vi "DefenderNormal.vi"(1 "Atacando contra?":bool=TRUE, 3 "AI Parameters":T1={"GotoKick"={"Dist do cone a frente"=150.0, "attacker farback"=1500.0, "Perto"=300.0, "min dist to kick"=150.0, "kick eps"=0.05, "Time to transition"=0.0}, "Attacker"={"CC chute"=0.09, "CC passe"=0.045, "Kick Force"=100.0, "D ball-robot Kick"=200.0, "D ball-robot Pass"=0.3}, "Defender"={"D max"=1700.0, "Vel p/ robô av"=1000.0, "Kick Force"=100.0, "D atk-def"=0.0, "D farback"=0.0}, "Timeout"={"Field/v in x"=6.0, "Dist Robots"=300, "Dist up in y"=300}, "Pose Striker"={"dist"=200.0, "Numeric"=-4.0, "dist 2"=200.0}, "Dist Stop"=300.0, "Distance when ball out"=200, "D central gap "=150.0, "T pass"=0.0, "Force ++"=0.0, "range kick"=0.0} {"D central gap" format="%#_13g"; "Dist Stop" format="%#_13g"; "Pose Striker"."Numeric" format="%#_13g"; "Defender"."Kick Force" format="%#_13g"; "Defender"."Vel p/ robô av" format="%#_13g"; "Attacker"."D ball-robot Kick" format="%#_13g"; "Attacker"."Kick Force" format="%#_13g"; "Attacker"."CC passe" format="%#_13g"; "Attacker"."CC chute" format="%#_13g"; "GotoKick"."kick eps" format="%#_13g"; "GotoKick"."min dist to kick" format="%#_13g"; "GotoKick"."Perto" format="%#_13g"; "GotoKick"."attacker farback" format="%#_13g"; "GotoKick"."Dist do cone a frente" format="%#_13g"}, 4 "IA State Input 2":T2={"our_robots"=[], "enemy_robots"=[], "balls"=[], "geometry"={"line_width"=0, "field_length"=0, "field_width"=0, "boundary_width"=0, "referee_width"=0, "goal_width"=0, "goal_depth"=0, "goal_wall_width"=0, "center_circle_radius"=0, "defense_radius"=0, "defense_stretch"=0, "free_kick_from_defense_dist"=0, "penalty_spot_from_field_line_dist"=0, "penalty_line_from_spot_dist"=0}, "IA Judge"={"stage"="", "command"="", "our_goalie_id"=0.0, "enemy_goalie_id"=0.0, "command enum"=enum."Halt", "Time"=enum."Azul"}, "Received Timestamp"=timestamp(0 s since 1904-01-01), "Events"={"Touch"=FALSE, "Ball out"=FALSE, "id touch"=0.0, "Ball out of \nVision"=FALSE, "Ball inside \nGoalie area"=FALSE, "Robot not responding"=FALSE, "Robots responding status"=[1.0, 1.0, 1.0, 1.0, 1.0, 1.0], "Enemy Ball \nPossession"=FALSE, "Pass State"=FALSE, "id end of pass"=0.0, "Kick"=FALSE, "Id ini Possession"=0.0, "Ball Possesion"=FALSE, "Id Possesion"=0.0}}, 5 "Stop?":bool, 6 "Defensores":u32[](array[numeric]), 7 "total":i32, 8 "Field defense":dbl[](array[numeric]), 9 "Field Size in":T7, 10 "balls":T6[](array[typedef]), 11 "Our Robot in":T3={"id"=0, "function"=enum."Attacker", "x"=0.0, "y"=0.0, "orientation"=0.0, "v_tangent"=0.0, "v_normal"=0.0, "v_ang"=0.0, "kick_x"=0.0, "kick_z"=0.0, "dribble"=FALSE, "Timestamp"=timestamp(0 s since 1904-01-01), "dest_x"=0.0, "dest_y"=0.0, "dest_orientation"=0.0, "estimatives"={"est_v_tangent"=0.0, "est_v_normal"=0.0, "est_vx"=0.0, "est_vy"=0.0, "Pos Robot Est"=[]}, "dest_x_kick"=0.0, "dest_y_kick"=0.0, "Gap Coord"=[], "States"=enum."GoToTangent"}) -> (2 "Robot out":T3={"id"=0, "function"=enum."Attacker", "x"=0.0, "y"=0.0, "orientation"=0.0, "v_tangent"=0.0, "v_normal"=0.0, "v_ang"=0.0, "kick_x"=0.0, "kick_z"=0.0, "dribble"=FALSE, "Timestamp"=timestamp(0 s since 1904-01-01), "dest_x"=0.0, "dest_y"=0.0, "dest_orientation"=0.0, "estimatives"={"est_v_tangent"=0.0, "est_v_normal"=0.0, "est_vx"=0.0, "est_vy"=0.0, "Pos Robot Est"=[]}, "dest_x_kick"=0.0, "dest_y_kick"=0.0, "Gap Coord"=[], "States"=enum."GoToTangent"})   [LabVIEW 2016]
uses:
  Core/AI Robot.ctl
  Functions Enum.ctl
  AttackerStates.ctl
  Core/AI Ball.ctl
  Core/Field Size.ctl
  Core/AI Input.ctl
  Core/AI Judge.ctl
  Command Enum.ctl
  Util/Events/Events.ctl
  AI Parameters.ctl
  <vilib>/Analysis/_algsub.llb/Real Vector Norm.vi
  <vilib>/Analysis/NI_AALPro.lvlib
panel:
  in  "element":dbl=-2000.0 format="%#_13g"
  in  "dist to defender\nattacker evasion":dbl=200.0
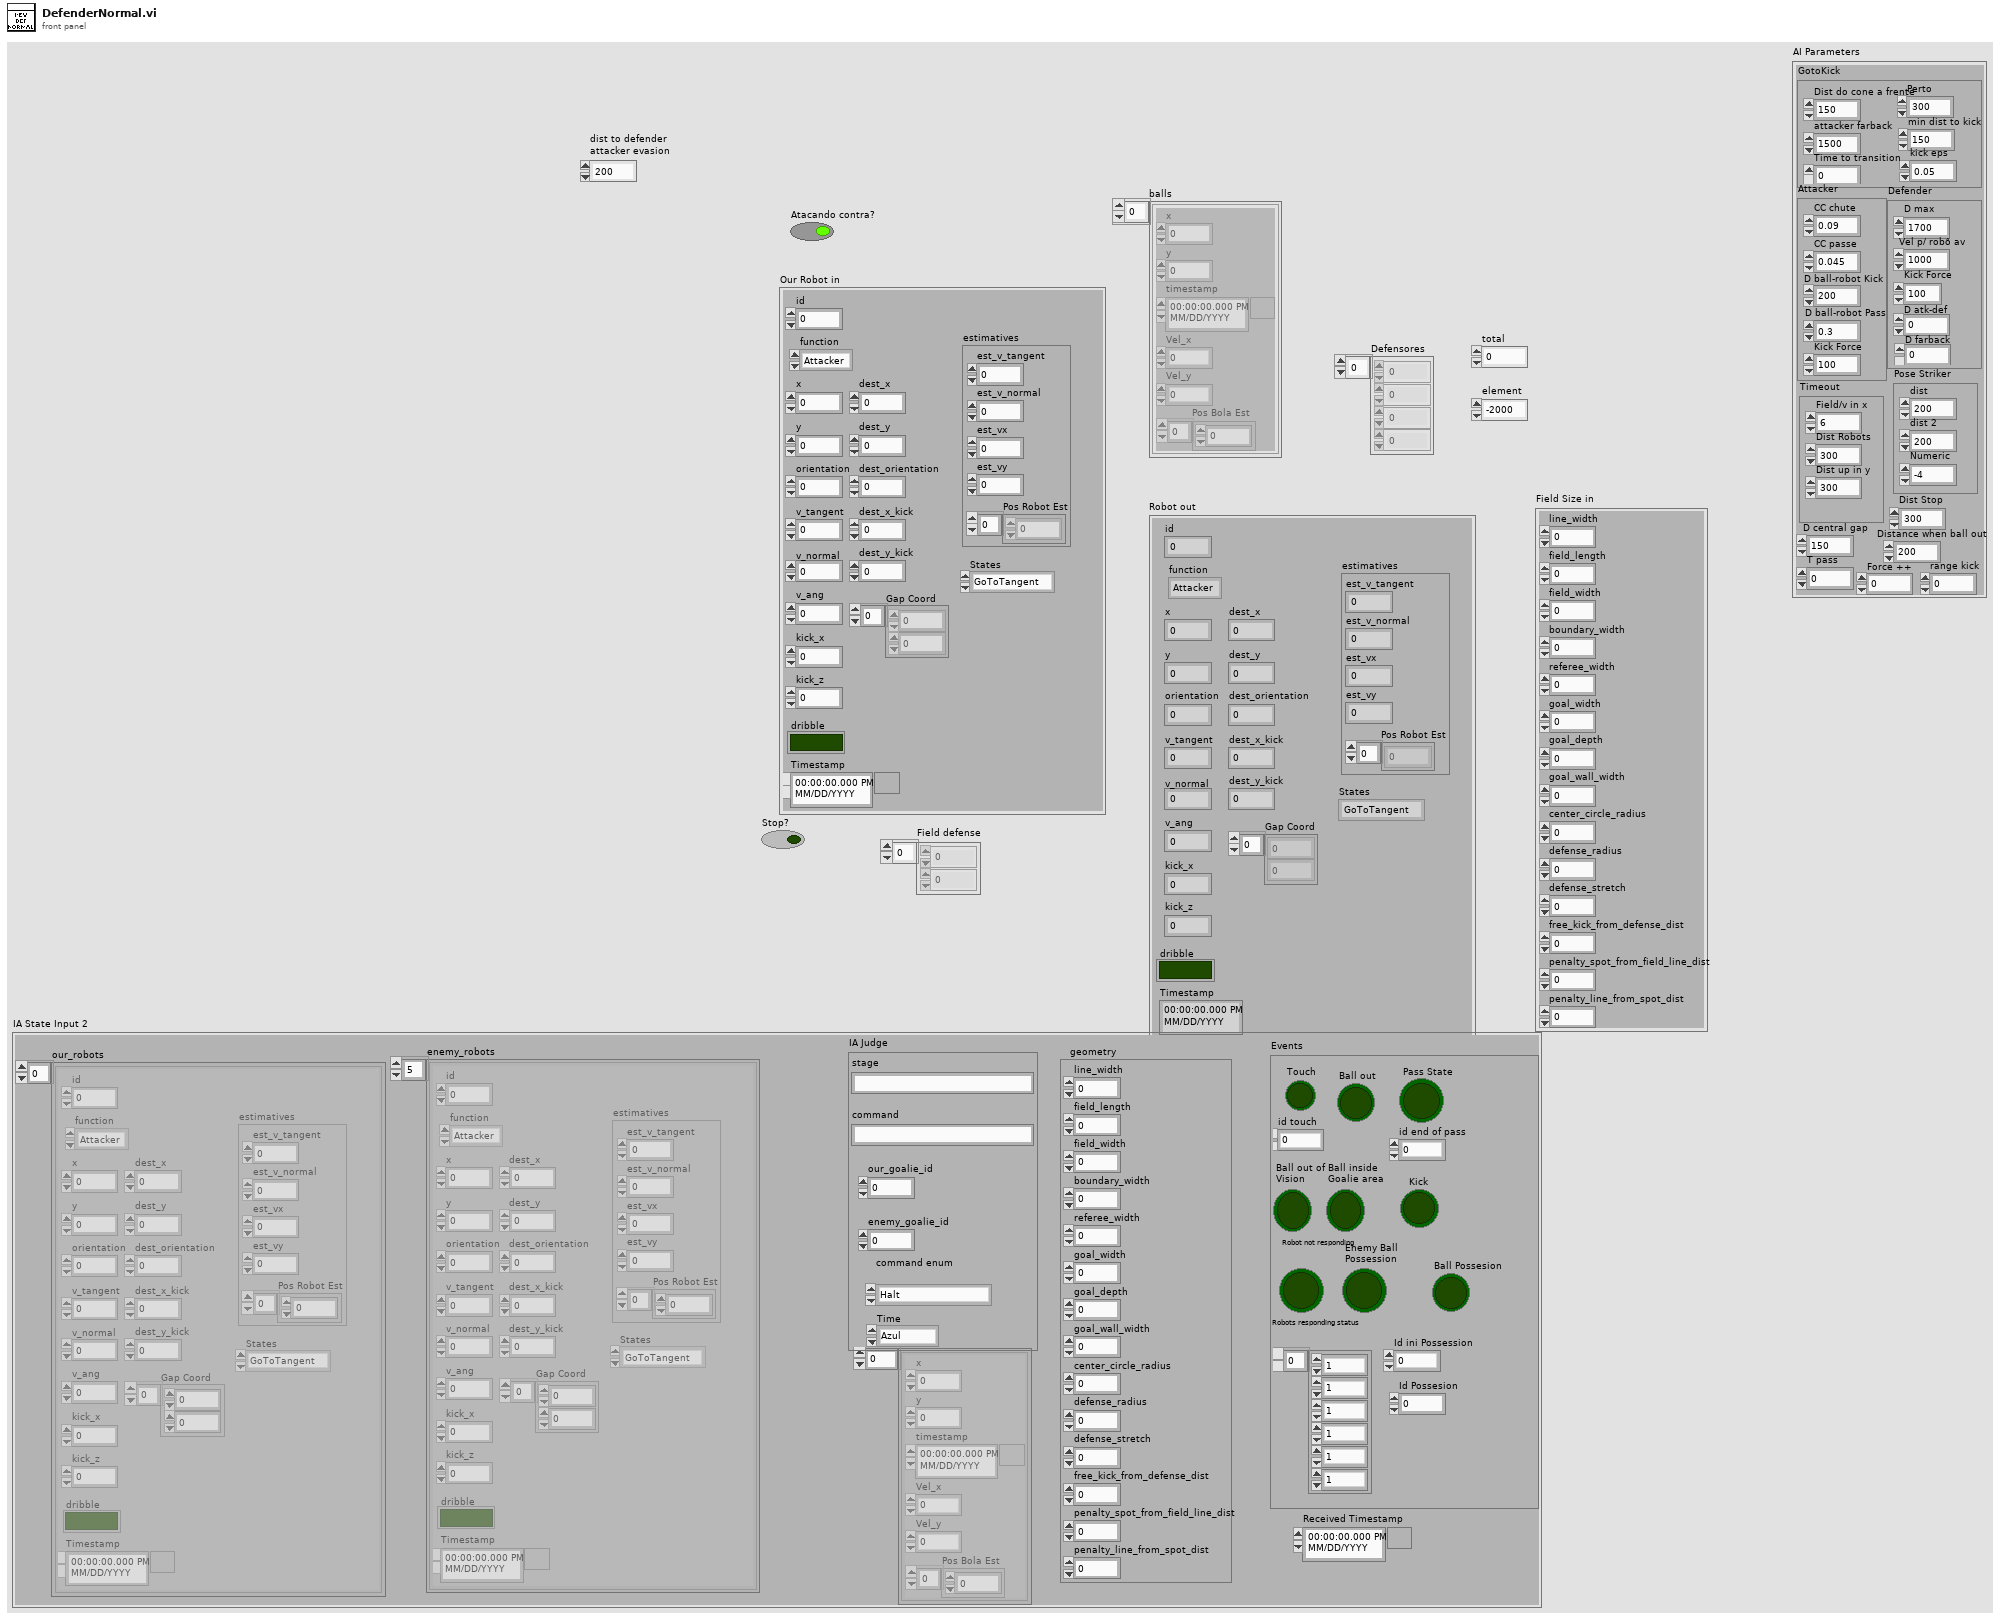
[diagram p1: front panel]
types:
  T1 = typedef "AI Parameters.ctl" = cluster{"GotoKick":cluster{"Dist do cone a frente":dbl, "attacker farback":dbl, "Perto":dbl, "min dist to kick":dbl, "kick eps":dbl, "Time to transition":dbl}, "Attacker":cluster{"CC chute":dbl, "CC passe":dbl, "Kick Force":dbl, "D ball-robot Kick":dbl, "D ball-robot Pass":dbl}, "Defender":cluster{"D max":dbl, "Vel p/ robô av":dbl, "Kick Force":dbl, "D atk-def":dbl, "D farback":dbl}, "Timeout":cluster{"Field/v in x":dbl, "Dist Robots":u32, "Dist up in y":u32}, "Pose Striker":cluster{"dist":dbl, "Numeric":dbl, "dist 2":dbl}, "Dist Stop":dbl, "Distance when ball out":i32, "D central gap ":dbl, "T pass":dbl, "Force ++":dbl, "range kick":dbl}
  T2 = typedef "AI Input.ctl" = cluster{"our_robots":T3[], "enemy_robots":T3[], "balls":T6[], "geometry":T7, "IA Judge":T8, "Received Timestamp":timestamp, "Events":T10}
  T3 = typedef "AI Robot.ctl" = cluster{"id":u32, "function":T4, "x":dbl, "y":dbl, "orientation":dbl, "v_tangent":dbl, "v_normal":dbl, "v_ang":dbl, "kick_x":dbl, "kick_z":dbl, "dribble":bool, "Timestamp":timestamp, "dest_x":dbl, "dest_y":dbl, "dest_orientation":dbl, "estimatives":cluster{"est_v_tangent":dbl, "est_v_normal":dbl, "est_vx":dbl, "est_vy":dbl, "Pos Robot Est":dbl[]}, "dest_x_kick":dbl, "dest_y_kick":dbl, "Gap Coord":dbl[], "States":T5}
  T4 = typedef "Functions Enum.ctl" = enum16{"Attacker", "Goalie", "Defender", "Striker", "Goto 0", "Dummy", "Kicker", "ZigZag"}
  T5 = typedef "AttackerStates.ctl" = enum16{"Pass", "GoToTangent", "BallGetting", "GoToKick", ""}
  T6 = typedef "AI Ball.ctl" = cluster{"x":dbl, "y":dbl, "timestamp":timestamp, "Vel_x":dbl, "Vel_y":dbl, "Pos Bola Est":dbl[]}
  T7 = typedef "Field Size.ctl" = cluster{"line_width":u32, "field_length":u32, "field_width":u32, "boundary_width":u32, "referee_width":u32, "goal_width":u32, "goal_depth":u32, "goal_wall_width":u32, "center_circle_radius":u32, "defense_radius":u32, "defense_stretch":u32, "free_kick_from_defense_dist":u32, "penalty_spot_from_field_line_dist":u32, "penalty_line_from_spot_dist":u32}
  T8 = typedef "AI Judge.ctl" = cluster{"stage":string, "command":string, "our_goalie_id":dbl, "enemy_goalie_id":dbl, "command enum":T9, "Time":enum16{"Azul", "Amarelo"}}
  T9 = typedef "Command Enum.ctl" = enum16{"Halt", "Stop", "Force Start", "PKA Normal Start", "Prepare Kickoff Ally", "PKE Normal Start", "Prepare Kickoff Enemy", "Prepare Penalty Ally", "PPA Normal Start", "Prepare Penalty Enemy", "PPE Normal Start", "Direct Free Enemy", "Direct Free Ally", "Indirect Free Enemy", "Indirect Free Ally", "Timeout Enemy", "Timeout Ally", "Goal Enemy", "Goal Ally", "Ball Placement Enemy", "Ball Placement Ally", "Normal Half Time", "Extra Time Break", "Extra Half Time", "None", "Post Game"}
  T10 = typedef "Events.ctl" = cluster{"Touch":bool, "Ball out":bool, "id touch":dbl, "Ball out of \nVision":bool, "Ball inside \nGoalie area":bool, "Robot not responding":bool, "Robots responding status":dbl[], "Enemy Ball \nPossession":bool, "Pass State":bool, "id end of pass":dbl, "Kick":bool, "Id ini Possession":dbl, "Ball Possesion":bool, "Id Possesion":dbl}
  T11 = cluster{"D max":dbl, "Vel p/ robô av":dbl, "Kick Force":dbl, "D atk-def":dbl, "D farback":dbl}
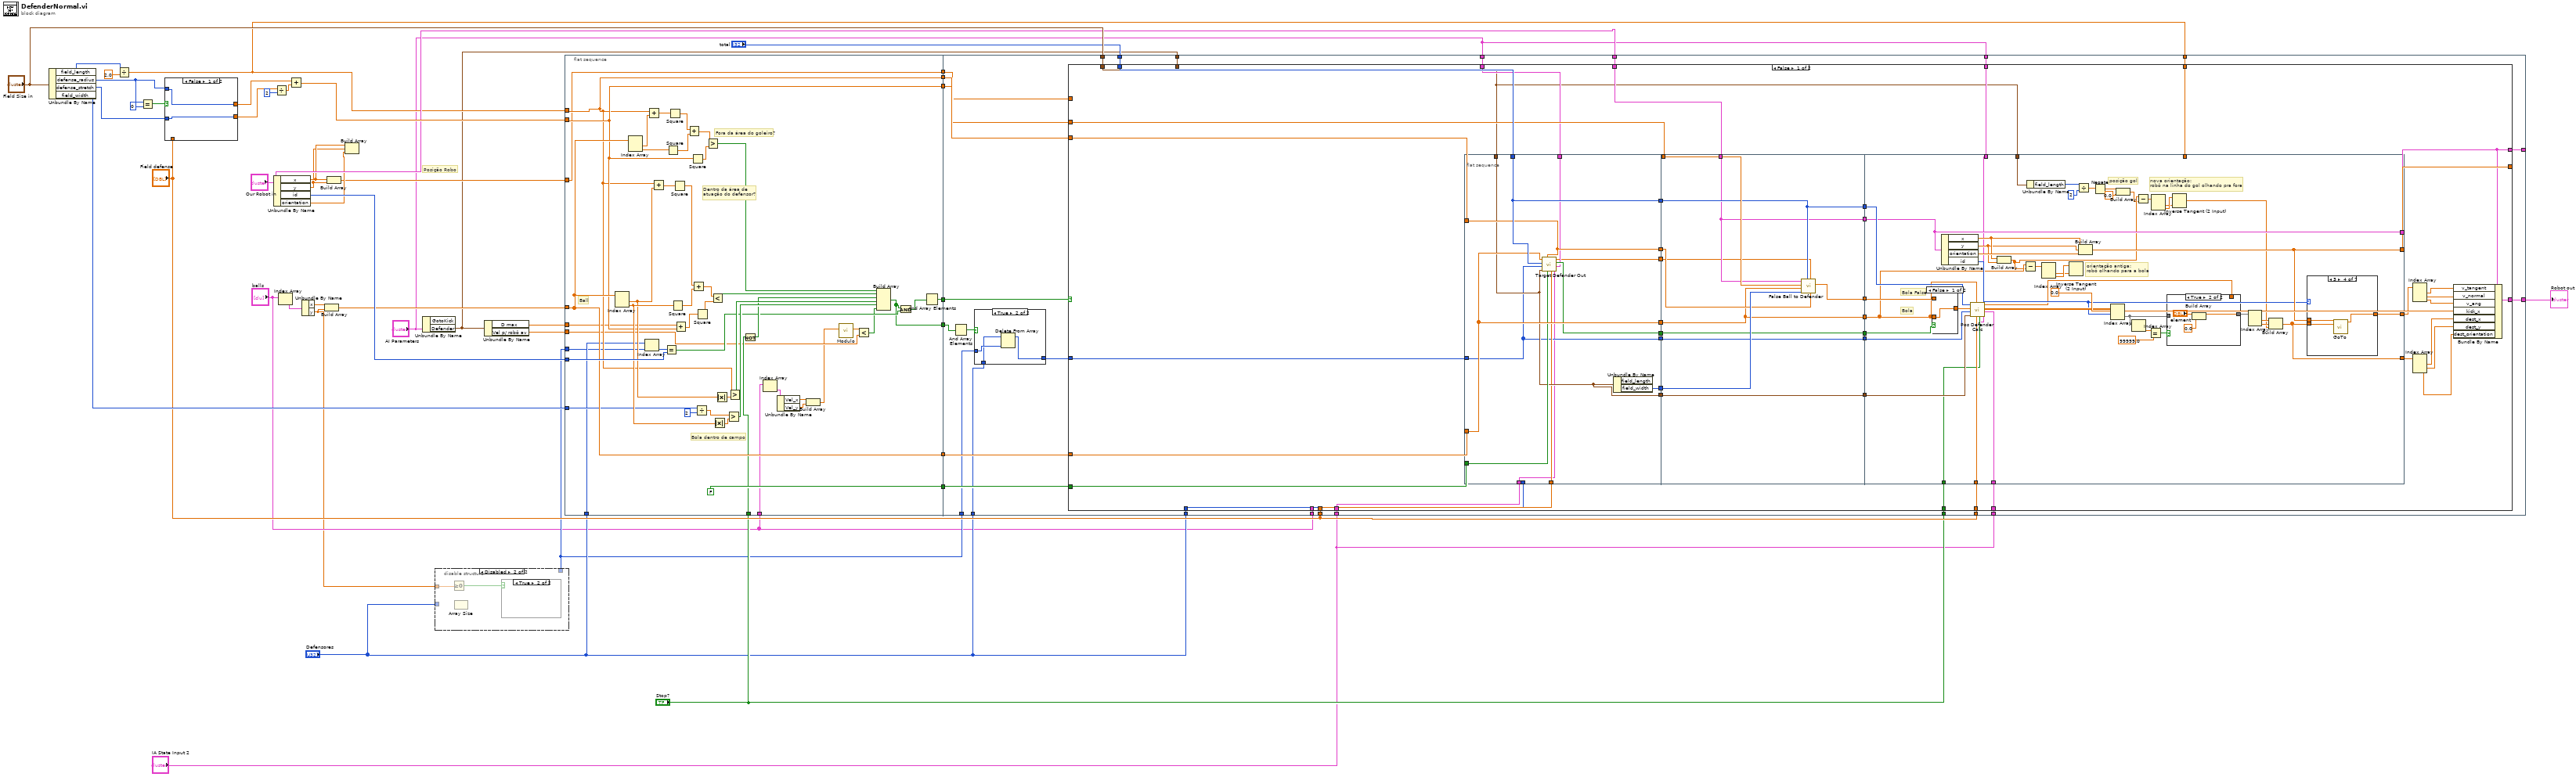
[diagram p0: block diagram]
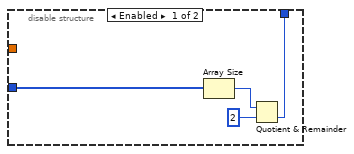
[diagram p2: hidden frame]
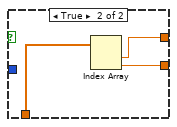
[diagram p4: hidden frame]
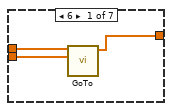
[diagram p7: hidden frame]
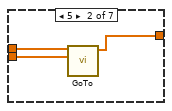
[diagram p8: hidden frame]
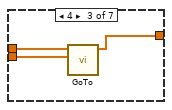
[diagram p9: hidden frame]
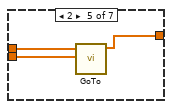
[diagram p10: hidden frame]
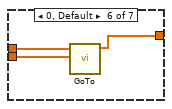
[diagram p11: hidden frame]
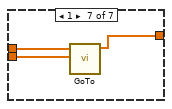
[diagram p12: hidden frame]
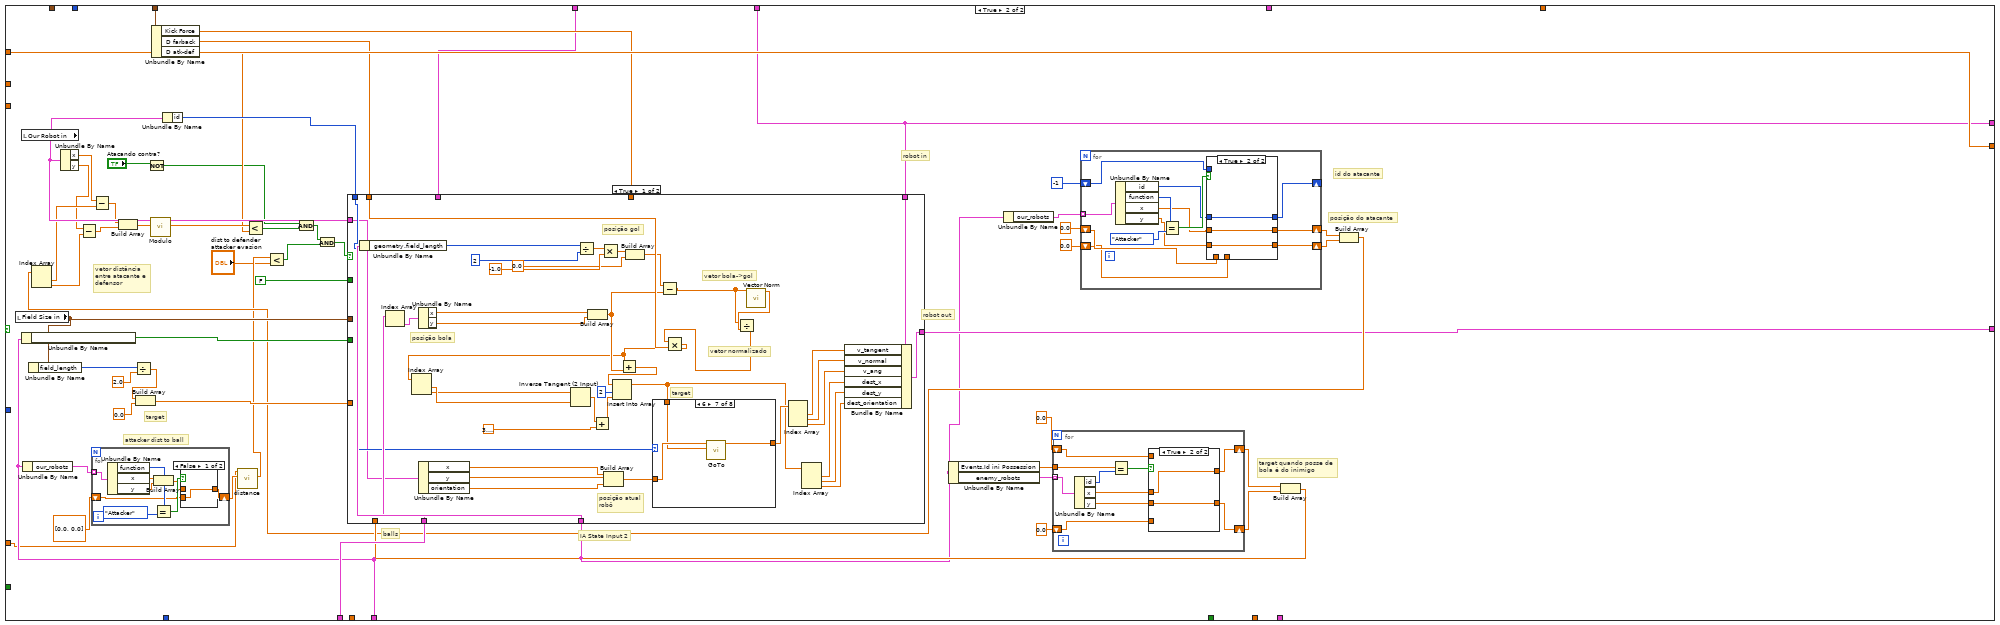
[diagram p14: hidden frame]
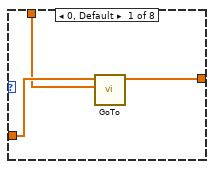
[diagram p16: hidden frame]
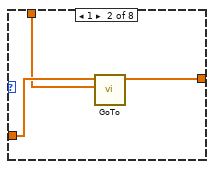
[diagram p17: hidden frame]
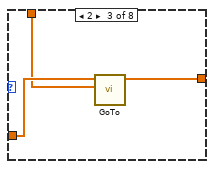
[diagram p18: hidden frame]
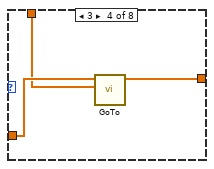
[diagram p19: hidden frame]
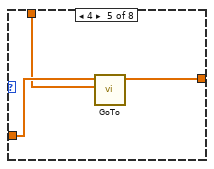
[diagram p20: hidden frame]
diagram:
  # "Posição Robo"
  n1 = Unbundle By Name("Field Size in") -> ("field_length"=w38:u32, "defense_radius"=w20:u32, "defense_stretch"=w19:u32, "field_width"=w35:u32)
  n2 = Divide(x=w38, y=2.0) -> (x/y=w11:dbl)
  n3 = Equal?(x=w20, y=u32 0) -> (x = y?=w18:bool)
  n4 = case shown="False" w18 {
    tunnel: [w45 w48] -> w17
    tunnel: w20 -> [w45 _]
    tunnel: w19 -> [w44 _]
    tunnel: [w44 w47] -> w16
    tunnel: "Field defense" -> [_ w46]
    frame False {
    }
    frame True {
      n5 = Index Array(array=w46) -> (element #1=w48:dbl, element #2=w47:dbl)  [unwired: 2 in]
    }
  }
  n6 = Unbundle By Name("Our Robot in") -> ("x"=w32:dbl, "y"=w31:dbl, "id"=w36:u32, "orientation"=w30:dbl)
  n7 = Divide(x=w16, y=u32 2) -> (x/y=w42:dbl)
  n8 = Index Array(array="balls") -> (element=w43:T6)  [unwired: 1 in]
  n9 = Add(x=w17, y=w42) -> (x+y=w37:dbl)
  n10 = Unbundle By Name(w43) -> ("x"=w40:dbl, "y"=w1:dbl)
  n11 = Build Array(w40, w1) -> (w12:dbl[])
  n12 = Build Array(w32, w31) -> (w13:dbl[])
  n13 = Build Array(w32, w31, w30) -> ()  [unwired: 1 out]
  n14 = Unbundle By Name("AI Parameters") -> ("Defender"=w4:T11)  [unwired: 1 out]
  n15 = disable-structure shown="Disabled" {
    disable-tunnel: "Defensores" -> [w50 _]
    disable-tunnel: [w49 _] -> w9
    disable-tunnel: w1 -> [_ w54]
    frame Enabled {
      n16 = Array Size(array=w50) -> (size(s)=w52:i32)
      n17 = Quotient & Remainder(x=w52, y=2) -> (floor(x/y)=w49:i32)  [unwired: 1 out]
    }
    frame Disabled {
      n18 = Greater Or Equal To 0?(x=w54) -> (x >= 0?=w53:bool)
      n19 = Array Size() -> ()  [unwired: 1 in, 1 out]
      n20 = case shown="True" w53 {
        frame False {
        }
        frame True {
        }
      }
    }
  }
  n21 = Unbundle By Name(w4) -> ("D max"=w6:dbl, "Vel p/ robô av"=w5:dbl)
  n22 = flat-sequence {
    tunnel: w37 -> [w74]
    tunnel: w11 -> [w73]
    tunnel: w12 -> [w89]
    tunnel: w13 -> [w72]
    tunnel: [w89] -> w29
    tunnel: [w94] -> w28
    tunnel: w36 -> [w93]
    tunnel: w35 -> [w80]
    tunnel: [FALSE ("Target Fora")] -> w27
    tunnel: [w73] -> w26
    tunnel: [w74] -> w25
    tunnel: [w72] -> w24
    tunnel: "Defensores" -> [w70]
    tunnel: "Stop?" -> [w69]
    tunnel: w9 -> [w68]
    tunnel: [w64] -> w8
    tunnel: "balls" -> [w63]
    tunnel: w6 -> [w60]
    tunnel: w5 -> [w59]
    tunnel: "total" -> [w129]
    tunnel: [w128] -> w22
    tunnel: w29 -> [w127]
    tunnel: w28 -> [w126]
    tunnel: w27 -> [w125]
    tunnel: w26 -> [w123]
    tunnel: "Field Size in" -> [w124]
    tunnel: "Our Robot in" -> [w122]
    tunnel: w25 -> [w121]
    tunnel: [w120] -> _
    tunnel: w24 -> [w119]
    tunnel: "Field defense" -> [w118]
    tunnel: "Field defense" -> [w117]
    tunnel: "Defensores" -> [w116]
    tunnel: "IA State Input 2" -> [w115]
    tunnel: "balls" -> [w114]
    tunnel: "Stop?" -> [w113]
    tunnel: w11 -> [w112]
    tunnel: "Defensores" -> [w110]
    tunnel: w9 -> [w111]
    tunnel: w8 -> [w109]
    tunnel: w4 -> [w106]
    tunnel: "AI Parameters" -> [w105]
    tunnel: "AI Parameters" -> [w104]
    tunnel: "IA State Input 2" -> [w103]
    frame #0 {
      # "Bola dentro de campo"
      # "Dentro da área de \natuação do defensor?"
      # "Fora da área do goleiro?"
      # "Ball"
      n23 = Index Array(array=w89) -> (element #1=w77:dbl, element #2=w81:dbl)  [unwired: 2 in]
      n24 = Index Array(array=w89) -> (element #1=w95:dbl, element #2=w97:dbl)  [unwired: 2 in]
      n25 = Index Array(array=w70, index=w68) -> (element=w71:u32)
      n26 = Add(x=w73, y=w95) -> (x+y=w96:dbl)
      n27 = Add(x=w73, y=w77) -> (x+y=w90:dbl)
      n28 = Equal?(x=w71, y=w93) -> (x = y?=w66:bool)
      n29 = Square(x=w97) -> (x^2=w99:dbl)
      n30 = Square(x=w96) -> (x^2=w98:dbl)
      n31 = Square(x=w81) -> (x^2=w92:dbl)
      n32 = Square(x=w90) -> (x^2=w91:dbl)
      n33 = Add(x=w60, y=w74) -> (x+y=w76:dbl)
      n34 = Add(x=w98, y=w99) -> (x+y=w100:dbl)
      n35 = Square(x=w74) -> (x^2=w101:dbl)
      n36 = Add(x=w91, y=w92) -> (x+y=w86:dbl)
      n37 = Divide(x=w80, y=u32 2) -> (x/y=w83:dbl)
      n38 = Square(x=w76) -> (x^2=w88:dbl)
      n39 = Greater?(x=w100, y=w101) -> (0:w102:bool)
      n40 = Less?(x=w86, y=w88) -> (x < y?=w87:bool)
      n41 = Absolute Value(x=w81) -> (abs(x)=w82:dbl)
      n42 = Absolute Value(x=w77) -> (abs(x)=w85:dbl)
      n43 = Greater?(x=w83, y=w82) -> (0:w78:bool)
      n44 = Greater?(x=w73, y=w85) -> (0:w84:bool)
      n45 = Not(x=w69) -> (.not. x?=w67:bool)
      n46 = Index Array(array=w63) -> (element=w58:T6)  [unwired: 1 in]
      n47 = Unbundle By Name(w58) -> ("Vel_x"=w57:dbl, "Vel_y"=w56:dbl)
      n48 = Build Array(w57, w56) -> (w55:dbl[])
      n49 = call "Modulo.vi"("2D vector"=w55) -> ("Modulo"=w61:dbl)  [unwired: 10 in]
      n50 = Less?(x=w61, y=w59) -> (x < y?=w62:bool)
      n51 = Build Array(w102, w87, w67, w84, w78, w62) -> (w64:bool[])
      n52 = And(x=w64, y=w66) -> (x .and. y?=w65:bool[])
      n53 = And Array Elements(Boolean array=w65) -> (logical AND=w94:bool)
    }
    frame #1 {
      n54 = And Array Elements(Boolean array=w109) -> (logical AND=w108:bool)
      n55 = case shown="True" w108 {
        tunnel: w111 -> [_ w133]
        tunnel: w110 -> [w130 w132]
        tunnel: [w130 w131] -> w107
        frame False {
        }
        frame True {
          n56 = Delete From Array(array=w132, index=w133) -> (array with subset deleted=w131:u32[])  [unwired: 1 in, 1 out]
        }
      }
      n57 = case shown="False" w126 {
        tunnel: w129 -> [w176 _]
        tunnel: [w171 w286] -> w128
        tunnel: w127 -> [w170 w276]
        tunnel: w125 -> [w168 _]
        tunnel: w123 -> [w167 _]
        tunnel: w124 -> [w134 _]
        tunnel: w122 -> [w166 w287]
        tunnel: w121 -> [w165 _]
        tunnel: [w151 w324] -> _
        tunnel: [w150 w287] -> w120
        tunnel: w119 -> [_ w324]
        tunnel: w118 -> [w149 _]
        tunnel: w117 -> [w148 _]
        tunnel: w116 -> [w147 _]
        tunnel: w115 -> [w137 w280]
        tunnel: w114 -> [_ w323]
        tunnel: w113 -> [w146 _]
        tunnel: w112 -> [w145 _]
        tunnel: w107 -> [w142 _]
        tunnel: w106 -> [_ w306]
        tunnel: w105 -> [w136 w304]
        tunnel: w104 -> [w139 _]
        tunnel: w103 -> [w138 _]
        frame False {
          n58 = flat-sequence {
            tunnel: w176 -> [w188]
            tunnel: [w189] -> w177
            tunnel: w170 -> [w187]
            tunnel: [w188] -> w169
            tunnel: w168 -> [w185]
            tunnel: w167 -> [w186]
            tunnel: w134 -> [w183]
            tunnel: [w187] -> w164
            tunnel: [w186] -> w163
            tunnel: [w184] -> w159
            tunnel: [w181] -> w156
            tunnel: [w183] -> w154
            tunnel: w148 -> [w182]
            tunnel: w147 -> [_]
            tunnel: w142 -> [w181]
            tunnel: w137 -> [w180]
            tunnel: w136 -> [w179]
            tunnel: [w178] -> w135
            tunnel: w177 -> [w200]
            tunnel: w169 -> [w194]
            tunnel: w166 -> [w191]
            tunnel: w165 -> [w199]
            tunnel: w164 -> [w196]
            tunnel: w163 -> [w198]
            tunnel: [w197] -> w162
            tunnel: [w196] -> w161
            tunnel: [w195] -> w160
            tunnel: w159 -> [w195]
            tunnel: [w194] -> w158
            tunnel: [w193] -> w157
            tunnel: w156 -> [w193]
            tunnel: [w192] -> w155
            tunnel: w154 -> [w192]
            tunnel: [w191] -> w153
            tunnel: w135 -> [w190]
            tunnel: [w236] -> w152
            tunnel: [w232] -> w150
            tunnel: w162 -> [w235]
            tunnel: w161 -> [w223]
            tunnel: w160 -> [w213]
            tunnel: w158 -> [w234]
            tunnel: w157 -> [w233]
            tunnel: w155 -> [w231]
            tunnel: w153 -> [w232]
            tunnel: [w227] -> w151
            tunnel: w149 -> [w225]
            tunnel: w146 -> [w224]
            tunnel: w145 -> [_]
            tunnel: [w217] -> w144
            tunnel: w139 -> [w215]
            tunnel: w138 -> [w214]
            tunnel: w134 -> [w212]
            frame #0 {
              n59 = call "Target Defender Out.vi"("IA State Input"=w180, "AI Parameters"=w179, "Field defense"=w182, "Target Fora in"=w185, "Campo/2"=w186, "Field Size in"=w183, "Defensores"=w181, "total"=w188, "Ball"=w187) -> ("Target Fora out"=w184:bool, "Central Position"=w178:dbl[])  [unwired: 1 in]
              n60 = Unbundle By Name(w183) -> ("field_width"=w189:u32)  [unwired: 1 out]
            }
            frame #1 {
              n61 = call "False Ball to Defender.vi"("Campo/2"=w198, "Central Position"=w190, "field_width"=w200, "total"=w194, "Bola"=w196, "raio da área \ndo goleiro"=w199, "Our Robot in"=w191) -> ("Bola Falsa"=w197:dbl[])  [unwired: 4 in]
            }
            frame #2 {
              # "nova orientação:\nrobô na linha do gol olhando pra fora"
              # "orientação antiga:\nrobô olhando para a bola"
              # "posição gol"
              # "Bola"
              # "Bola Falsa"
              n62 = case shown="False" w213 {
                tunnel: [w269 w270] -> w243
                tunnel: w235 -> [_ w270]
                tunnel: w223 -> [w269 _]
                frame False {
                }
                frame True {
                }
              }
              n63 = Unbundle By Name(w232) -> ("x"=w241:dbl, "y"=w240:dbl, "orientation"=w242:dbl, "id"=w226:u32)
              n64 = call "Pos Defender Calc.vi"("IA State Input"=w214, "AI Parameters"=w215, "Stop?"=w224, "Field defense"=w225, "Real Ball"=w223, "Field Size in"=w231, "Defensores"=w233, "Ball"=w243, "total"=w234) -> ("Posição dos Defensores"=w230:dbl[][], "Central Position"=w216:dbl[])  [unwired: 1 in]
              n65 = Build Array(w241, w240) -> (w206:dbl[])
              n66 = Subtract(x=w223, y=w206) -> (x-y=w239:dbl[])
              n67 = Unbundle By Name(w212) -> ("field_length"=w211:u32)
              n68 = Index Array(array=w239) -> (element #1=w237:dbl, element #2=w238:dbl)  [unwired: 2 in]
              n69 = Inverse Tangent (2 Input)(1:w237, 2:w238) -> ()  [unwired: 1 out]
              n70 = Divide(x=w211, y=u32 2) -> (x/y=w209:dbl)
              n71 = Build Array(w241, w240, w242) -> (w227:dbl[])
              n72 = Negate(x=w209) -> (-x=w208:dbl)
              n73 = Index Array(array=w230, index (row)=w226) -> (element=w221:dbl[])  [unwired: 1 in]
              n74 = Build Array(w208, 0.0 ("element")) -> (w205:dbl[])
              n75 = Index Array(array=w221) -> (element=w220:dbl)  [unwired: 1 in]
              n76 = Subtract(x=w206, y=w205) -> (x-y=w204:dbl[])
              n77 = Equal?(x=w220, y=99999.0) -> (x = y?=w219:bool)
              n78 = Index Array(array=w204) -> (element #1=w202:dbl, element #2=w203:dbl)  [unwired: 2 in]
              n79 = case shown="True" w219 {
                tunnel: [w244 w246] -> w222
                tunnel: w221 -> [w244 _]
                tunnel: w216 -> [_ _]
                frame False {
                }
                frame True {
                  n80 = Build Array("element", 0.0 ("element")) -> (w246:dbl[])
                }
              }
              n81 = Inverse Tangent (2 Input)(1:w202, 2:w203) -> (0:w201:dbl)
              n82 = Index Array(array=w222) -> (element #1=w229:dbl, element #2=w228:dbl)  [unwired: 2 in]
              n83 = Build Array(w229, w228, w201) -> (w217:dbl[])
              n84 = case shown="3" w226 {
                tunnel: [w248 w251 w254 w257 w260 w263 w266] -> w236
                tunnel: w217 -> [w249 w253 w255 w258 w261 w264 w267]
                tunnel: w227 -> [w250 w252 w256 w259 w262 w265 w268]
                frame 6 {
                  n85 = call "GoTo.vi"("Target"=w249, "Position"=w250) -> ("Output\nVelocity"=w248:dbl[])  [unwired: 8 in, 1 out]
                }
                frame 5 {
                  n86 = call "GoTo.vi"("Target"=w253, "Position"=w252) -> ("Output\nVelocity"=w251:dbl[])  [unwired: 8 in, 1 out]
                }
                frame 4 {
                  n87 = call "GoTo.vi"("Target"=w255, "Position"=w256) -> ("Output\nVelocity"=w254:dbl[])  [unwired: 8 in, 1 out]
                }
                frame 3 {
                  n88 = call "GoTo.vi"("Target"=w258, "Position"=w259) -> ("Output\nVelocity"=w257:dbl[])  [unwired: 8 in, 1 out]
                }
                frame 2 {
                  n89 = call "GoTo.vi"("Target"=w261, "Position"=w262) -> ("Output\nVelocity"=w260:dbl[])  [unwired: 8 in, 1 out]
                }
                frame 0, Default {
                  n90 = call "GoTo.vi"("Target"=w264, "Position"=w265) -> ("Output\nVelocity"=w263:dbl[])  [unwired: 8 in, 1 out]
                }
                frame 1 {
                  n91 = call "GoTo.vi"("Target"=w267, "Position"=w268) -> ("Output\nVelocity"=w266:dbl[])  [unwired: 8 in, 1 out]
                }
              }
            }
          }
          n92 = Index Array(array=w152) -> (element #1=w174:dbl, element #2=w173:dbl, element #3=w172:dbl)  [unwired: 3 in]
          n93 = Index Array(array=w144) -> (element #1=w143:dbl, element #2=w141:dbl, element #3=w140:dbl)  [unwired: 3 in]
          n94 = Bundle By Name(cluster=w150, "v_tangent"=w174, "v_normal"=w173, "v_ang"=w172, "kick_x"=0.0, "dest_x"=w143, "dest_y"=w141, "dest_orientation"=w140) -> (w171:T3)
        }
        frame True {
          # "attacker dist to ball"
          # "robot in"
          # "vetor distância\nentre atacante e \ndefensor"
          # "posição do atacante"
          # "id do atacante"
          # "target quando posse de\nbola é do inimigo"
          # "target"
          # "balls"
          # "IA State Input 2"
          # "robot out"
          n95 = local read "Field Size in"() -> (w319:T7)
          n96 = local read "Our Robot in"() -> (w297:T3)
          n97 = Unbundle By Name(w280) -> ("Events.Enemy Ball \nPossession"=w314:bool)
          n98 = Unbundle By Name(w280) -> ("our_robots"=w279:T3[])
          n99 = Unbundle By Name(w319) -> ("field_length"=w318:u32)
          n100 = Unbundle By Name(w297) -> ("x"=w295:dbl, "y"=w293:dbl)
          n101 = for {
            tunnel: w279 -> [w333] mode=indexing
            shift-right: [w327] -> w277
            shift-left: dbl[] [0.0, 0.0] -> [w326]
            n102 = Unbundle By Name(w333) -> ("function"=w332:T4, "x"=w325:dbl, "y"=w329:dbl)
            n103 = Build Array(w325, w329) -> (w328:dbl[])
            n104 = Equal?(x=w332, y=Functions_Enum."Attacker") -> (x = y?=w330:bool)
            n105 = case shown="False" w330 {
              tunnel: w328 -> [_ w335]
              tunnel: [w334 w335] -> w327
              tunnel: w326 -> [w334 _]
              frame False {
              }
              frame True {
              }
            }
          }
          n106 = Divide(x=w318, y=2.0) -> (x/y=w316:dbl)
          n107 = Build Array(w316, 0.0) -> (w321:dbl[])
          n108 = Not(x="Atacando contra?") -> (.not. x?=w281:bool)
          n109 = Unbundle By Name(w306) -> ("Kick Force"=w305:dbl, "D farback"=w284:dbl, "D atk-def"=w285:dbl)
          n110 = Unbundle By Name(w297) -> ("id"=w322:u32)
          n111 = call "distance.vi"("target pos"=w277, "obj pos"=w276) -> ("sqrt(x)"=w275:dbl)  [unwired: 9 in]
          n112 = Less?(x=w275, y="dist to defender\nattacker evasion") -> (x < y?=w273:bool)
          n113 = Unbundle By Name(w280) -> ("Events.Id ini Possession"=w312:dbl, "enemy_robots"=w313:T3[])
          n114 = Unbundle By Name(w280) -> ("our_robots"=w303:T3[])
          n115 = for {
            tunnel: w313 -> [w538] mode=indexing
            tunnel: w312 -> [w536]
            shift-right: [w532] -> w311
            shift-left: 0.0 ("x") -> [w530]
            shift-right: [w531] -> w310
            shift-left: 0.0 ("y") -> [w529]
            n116 = Unbundle By Name(w538) -> ("id"=w537:u32, "x"=w534:dbl, "y"=w533:dbl)
            n117 = Equal?(x=w536, y=w537) -> (x = y?=w535:bool)
            n118 = case shown="True" w535 {
              tunnel: w534 -> [_ w542]
              tunnel: w533 -> [_ w541]
              tunnel: [w540 w542] -> w532
              tunnel: [w539 w541] -> w531
              tunnel: w530 -> [w540 _]
              tunnel: w529 -> [w539 _]
              frame False {
              }
              frame True {
              }
            }
          }
          n119 = for {
            tunnel: w303 -> [w522] mode=indexing
            shift-right: [w515] -> _
            shift-left: -1 -> [w514]
            shift-right: [w513] -> w299
            shift-left: 0.0 ("y") -> [w511]
            shift-right: [w512] -> w298
            shift-left: 0.0 ("y") -> [w510]
            n120 = Unbundle By Name(w522) -> ("id"=w518:u32, "function"=w521:T4, "x"=w517:dbl, "y"=w516:dbl)
            n121 = Equal?(x=w521, y=Functions_Enum."Attacker" ("x")) -> (x = y?=w519:bool)
            n122 = case shown="True" w519 {
              tunnel: w518 -> [_ w526]
              tunnel: w517 -> [_ w528]
              tunnel: w516 -> [_ w527]
              tunnel: [w524 w528] -> w513
              tunnel: [w523 w527] -> w512
              tunnel: [w525 w526] -> w515
              tunnel: w514 -> [w525 _]
              tunnel: w511 -> [w524 _]
              tunnel: w510 -> [w523 _]
              frame False {
              }
              frame True {
              }
            }
          }
          n123 = Build Array(w311, w310) -> (w307:dbl[])
          n124 = Build Array(w299, w298) -> (w296:dbl[])
          n125 = Index Array(array=w296) -> (element #1=w294:dbl, element #2=w292:dbl)  [unwired: 2 in]
          n126 = Subtract(x=w293, y=w292) -> (x-y=w290:dbl)
          n127 = Subtract(x=w295, y=w294) -> (x-y=w291:dbl)
          n128 = Build Array(w291, w290) -> (w289:dbl[])
          n129 = call "Modulo.vi"("2D vector"=w289) -> ("Modulo"=w288:dbl)  [unwired: 10 in]
          n130 = Less?(x=w288, y=w285) -> (x < y?=w283:bool)
          n131 = And(x=w281, y=w283) -> (x .and. y?=w272:bool)
          n132 = And(x=w272, y=w273) -> (x .and. y?=w271:bool)
          n133 = case shown="True" w271 {
            tunnel: w323 -> [w370 w413]
            tunnel: w322 -> [w365 w412]
            tunnel: w321 -> [_ w402]
            tunnel: w319 -> [_ w411]
            tunnel: FALSE -> [_ w410]
            tunnel: w314 -> [_ w404]
            tunnel: w307 -> [_ w403]
            tunnel: w305 -> [_ w409]
            tunnel: w304 -> [_ w408]
            tunnel: w280 -> [w371 w407]
            tunnel: w297 -> [w364 w406]
            tunnel: w287 -> [w348 _]
            tunnel: [w347 w405] -> w286
            tunnel: w284 -> [w345 _]
            frame True {
              # "target"
              # "posição atual\nrobô"
              # "vetor normalizado"
              # "vetor bola->gol"
              # "posição bola"
              # "posição gol"
              n134 = Unbundle By Name(w371) -> ("geometry.field_length"=w372:u32)
              n135 = Index Array(array=w370) -> (element=w376:T6)  [unwired: 1 in]
              n136 = Unbundle By Name(w376) -> ("x"=w342:dbl, "y"=w341:dbl)
              n137 = Unbundle By Name(w364) -> ("x"=w363:dbl, "y"=w362:dbl, "orientation"=w361:dbl)
              n138 = Divide(x=w372, y=u32 2) -> (x/y=w374:dbl)
              n139 = Build Array(w342, w341) -> (w338:dbl[])
              n140 = Multiply(x=w374, y=-1.0) -> (x*y=w344:dbl)
              n141 = Build Array(w363, w362, w361) -> (w360:dbl[])
              n142 = Build Array(w344, 0.0 ("element")) -> (w340:dbl[])
              n143 = Subtract(x=w340, y=w338) -> (x-y=w339:dbl[])
              n144 = call-poly <vilib>:"Vector Norm.vi"("Input Vector"=w339) -> ("norm"=w369:dbl)  [unwired: 9 in, 1 out]
              n145 = Divide(x=w339, y=w369) -> (x/y=w346:dbl[])
              n146 = Multiply(x=w346, y=w345) -> (x*y=w336:dbl[])
              n147 = Index Array(array=w336) -> (element #1=w368:dbl, element #2=w367:dbl)  [unwired: 2 in]
              n148 = Inverse Tangent (2 Input)(1:w368, 2:w367) -> (0:w359:dbl)
              n149 = Add(x=w359, y=3.141592653589793) -> (x+y=w357:dbl)
              n150 = Add(x=w336, y=w338) -> (x+y=w337:dbl[])
              n151 = Insert Into Array(array=w337, index=2, new element=w357) -> (w352:dbl[])
              n152 = case shown="6" w365 {
                tunnel: w360 -> [w379 w382 w385 w388 w391 w394 w397 w400]
                tunnel: w352 -> [w378 w381 w384 w387 w390 w393 w396 w399]
                tunnel: [w377 w380 w383 w386 w389 w392 w395 w398] -> w356
                frame 0, Default {
                  n153 = call "GoTo.vi"("Target"=w378, "Position"=w379) -> ("Output\nVelocity"=w377:dbl[])  [unwired: 8 in, 1 out]
                }
                frame 1 {
                  n154 = call "GoTo.vi"("Target"=w381, "Position"=w382) -> ("Output\nVelocity"=w380:dbl[])  [unwired: 8 in, 1 out]
                }
                frame 2 {
                  n155 = call "GoTo.vi"("Target"=w384, "Position"=w385) -> ("Output\nVelocity"=w383:dbl[])  [unwired: 8 in, 1 out]
                }
                frame 3 {
                  n156 = call "GoTo.vi"("Target"=w387, "Position"=w388) -> ("Output\nVelocity"=w386:dbl[])  [unwired: 8 in, 1 out]
                }
                frame 4 {
                  n157 = call "GoTo.vi"("Target"=w390, "Position"=w391) -> ("Output\nVelocity"=w389:dbl[])  [unwired: 8 in, 1 out]
                }
                frame 5 {
                  n158 = call "GoTo.vi"("Target"=w393, "Position"=w394) -> ("Output\nVelocity"=w392:dbl[])  [unwired: 8 in, 1 out]
                }
                frame 6 {
                  n159 = call "GoTo.vi"("Target"=w396, "Position"=w397) -> ("Output\nVelocity"=w395:dbl[])  [unwired: 8 in, 1 out]
                }
                frame 7 {
                  n160 = call "GoTo.vi"("Target"=w399, "Position"=w400) -> ("Output\nVelocity"=w398:dbl[])  [unwired: 8 in, 1 out]
                }
              }
              n161 = Index Array(array=w356) -> (element #1=w355:dbl, element #2=w354:dbl, element #3=w353:dbl)  [unwired: 3 in]
              n162 = Index Array(array=w352) -> (element #1=w351:dbl, element #2=w350:dbl, element #3=w349:dbl)  [unwired: 3 in]
              n163 = Bundle By Name(cluster=w348, "v_tangent"=w355, "v_normal"=w354, "v_ang"=w353, "dest_x"=w351, "dest_y"=w350, "dest_orientation"=w349) -> (w347:T3)
            }
            frame False {
              n164 = Select(t=w403, s=w404, f=w402) -> (s? t:f=w401:dbl[])
              n165 = case shown="2" w412 {
                tunnel: w406 -> [w424 w436 w448 w460 w472 w484 w496 w507]
                tunnel: w411 -> [w425 w437 w449 w461 w473 w485 w497 w505]
                tunnel: w413 -> [w423 w435 w447 w459 w471 w483 w495 w509]
                tunnel: w407 -> [w422 w434 w446 w458 w470 w482 w494 w508]
                tunnel: [w421 w433 w445 w457 w469 w481 w493 w506] -> w405
                tunnel: w410 -> [w420 w432 w444 w456 w468 w480 w492 w504]
                tunnel: w409 -> [w419 w431 w443 w455 w467 w479 w491 w503]
                tunnel: w408 -> [w418 w430 w442 w454 w466 w478 w490 w502]
                tunnel: w401 -> [w415 w427 w439 w451 w463 w475 w487 w499]
                frame 0, Default {
                  n166 = Unbundle By Name(w418) -> ("Attacker.D ball-robot Kick"=w417:dbl, "Attacker.CC chute"=w416:dbl)
                  n167 = call "GoToKick.vi"("goleiro?"=w420, "balls"=w423, "Robot in in"=w424, "Field Size in"=w425, "Target"=w415, "Defender"=TRUE, "D ball - robot"=w417, "AI Parameters"=w418, "Cone de chute"=w416, "Kick Force"=w419, "IA State Input in"=w422) -> ("Robot out"=w421:T3)  [unwired: 5 in, 3 out]
                }
                frame 2 {
                  n168 = Unbundle By Name(w430) -> ("Attacker.D ball-robot Kick"=w429:dbl, "Attacker.CC chute"=w428:dbl)
                  n169 = call "GoToKick.vi"("goleiro?"=w432, "balls"=w435, "Robot in in"=w436, "Field Size in"=w437, "Target"=w427, "Defender"=TRUE, "D ball - robot"=w429, "AI Parameters"=w430, "Cone de chute"=w428, "Kick Force"=w431, "IA State Input in"=w434) -> ("Robot out"=w433:T3)  [unwired: 5 in, 3 out]
                }
                frame 3 {
                  n170 = Unbundle By Name(w442) -> ("Attacker.D ball-robot Kick"=w441:dbl, "Attacker.CC chute"=w440:dbl)
                  n171 = call "GoToKick.vi"("goleiro?"=w444, "balls"=w447, "Robot in in"=w448, "Field Size in"=w449, "Target"=w439, "Defender"=TRUE, "D ball - robot"=w441, "AI Parameters"=w442, "Cone de chute"=w440, "Kick Force"=w443, "IA State Input in"=w446) -> ("Robot out"=w445:T3)  [unwired: 5 in, 3 out]
                }
                frame 4 {
                  n172 = Unbundle By Name(w454) -> ("Attacker.D ball-robot Kick"=w453:dbl, "Attacker.CC chute"=w452:dbl)
                  n173 = call "GoToKick.vi"("goleiro?"=w456, "balls"=w459, "Robot in in"=w460, "Field Size in"=w461, "Target"=w451, "Defender"=TRUE, "D ball - robot"=w453, "AI Parameters"=w454, "Cone de chute"=w452, "Kick Force"=w455, "IA State Input in"=w458) -> ("Robot out"=w457:T3)  [unwired: 5 in, 3 out]
                }
                frame 5 {
                  n174 = Unbundle By Name(w466) -> ("Attacker.D ball-robot Kick"=w465:dbl, "Attacker.CC chute"=w464:dbl)
                  n175 = call "GoToKick.vi"("goleiro?"=w468, "balls"=w471, "Robot in in"=w472, "Field Size in"=w473, "Target"=w463, "Defender"=TRUE, "D ball - robot"=w465, "AI Parameters"=w466, "Cone de chute"=w464, "Kick Force"=w467, "IA State Input in"=w470) -> ("Robot out"=w469:T3)  [unwired: 5 in, 3 out]
                }
                frame 6 {
                  n176 = Unbundle By Name(w478) -> ("Attacker.D ball-robot Kick"=w477:dbl, "Attacker.CC chute"=w476:dbl)
                  n177 = call "GoToKick.vi"("goleiro?"=w480, "balls"=w483, "Robot in in"=w484, "Field Size in"=w485, "Target"=w475, "Defender"=TRUE, "D ball - robot"=w477, "AI Parameters"=w478, "Cone de chute"=w476, "Kick Force"=w479, "IA State Input in"=w482) -> ("Robot out"=w481:T3)  [unwired: 5 in, 3 out]
                }
                frame 7 {
                  n178 = Unbundle By Name(w490) -> ("Attacker.D ball-robot Kick"=w489:dbl, "Attacker.CC chute"=w488:dbl)
                  n179 = call "GoToKick.vi"("goleiro?"=w492, "balls"=w495, "Robot in in"=w496, "Field Size in"=w497, "Target"=w487, "Defender"=TRUE, "D ball - robot"=w489, "AI Parameters"=w490, "Cone de chute"=w488, "Kick Force"=w491, "IA State Input in"=w494) -> ("Robot out"=w493:T3)  [unwired: 5 in, 3 out]
                }
                frame 1 {
                  n180 = Unbundle By Name(w502) -> ("Attacker.D ball-robot Kick"=w501:dbl, "Attacker.CC chute"=w500:dbl)
                  n181 = call "GoToKick.vi"("goleiro?"=w504, "balls"=w509, "Robot in in"=w507, "Field Size in"=w505, "Target"=w499, "Defender"=TRUE, "D ball - robot"=w501, "AI Parameters"=w502, "Cone de chute"=w500, "Kick Force"=w503, "IA State Input in"=w508) -> ("Robot out"=w506:T3)  [unwired: 5 in, 3 out]
                }
              }
            }
          }
        }
      }
    }
  }
  "Robot out" <- w22
